vi "Old Auto Sequence.vi"() -> ()   [LabVIEW 2014]
uses:
  TypeDefs/SRE Enum.ctl
  <vilib>/Rock Robotics/Network Tables/SD Read Number.vi
  Support Code/Robot Global Data.vi
panel:
  in  "Direction":dbl=1.25 format="%#_13g"
  in  "Set To":dbl=-135.0 format="%#_13g"
  in  "Angle":dbl=-155.0 format="%#_13g"
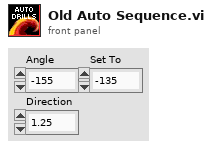
[diagram p1: front panel]
types:
  T1 = typedef "SRE Enum.ctl" = enum16{"Start", "Run", "End"}
  T2 = cluster{"Speed":dbl, "Direction":dbl, "Rotation":dbl}
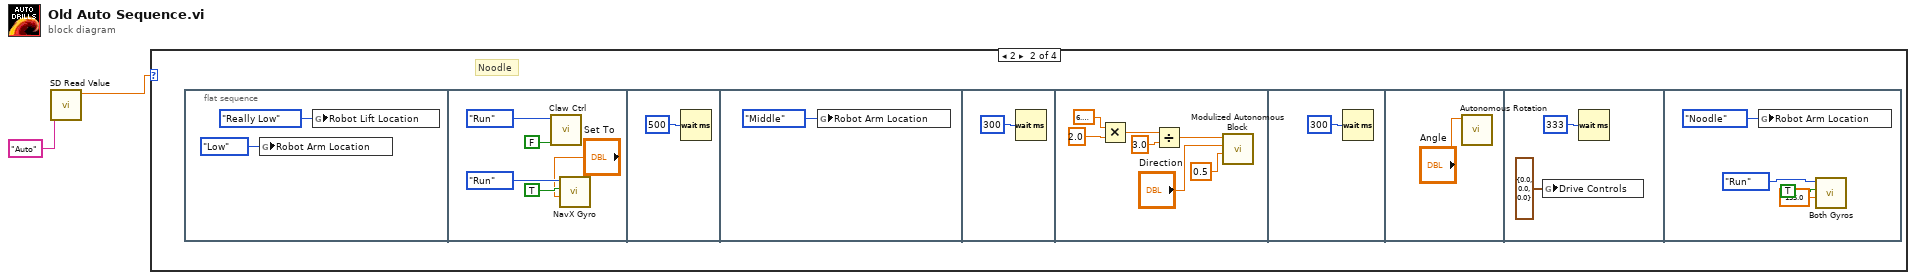
[diagram p0: block diagram]
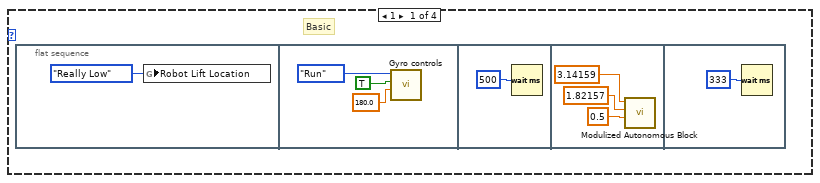
[diagram p2: hidden frame]
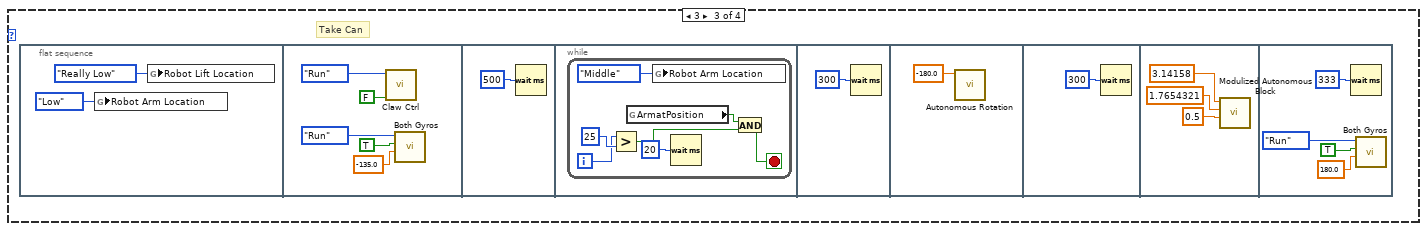
[diagram p3: hidden frame]
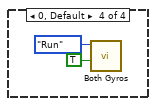
[diagram p4: hidden frame]
diagram:
  n1 = call-poly <vilib>:"SD Read Value.vi"("Name"="Auto") -> ("Numeric"=w1:dbl)  [unwired: 8 in, 2 out]
  n2 = case shown="2" w1 {
    frame 1 {
      # "Basic"
      n3 = flat-sequence {
        frame #0 {
          n4 = global write "Robot Global Data.vi" "Robot Lift Location"(enum16{"High", "Middle", "Low", "Really Low"}."Really Low" ("Robot Lift Location")) -> ()
        }
        frame #1 {
          n5 = call "Gyro controls.vi"("Set To"=180.0, "Reset"=TRUE, "Enum"=SRE_Enum."Run") -> ()  [unwired: 8 in, 1 out]
        }
        frame #2 {
          n6 = Wait (ms)(milliseconds to wait=u32 500) -> ()  [unwired: 1 out]
        }
        frame #3 {
          n7 = call "Modulized Autonomous Block.vi"("Power"=0.5, "run time in seconds"=1.82157 ("Direction"), "Direction"=3.14159) -> ()  [unwired: 8 in, 1 out]
        }
        frame #4 {
          n8 = Wait (ms)(milliseconds to wait=u32 333) -> ()  [unwired: 1 out]
        }
      }
    }
    frame 2 {
      # "Noodle"
      n9 = flat-sequence {
        frame #0 {
          n10 = global write "Robot Global Data.vi" "Robot Arm Location"(enum16{"High", "Middle", "Low", "Noodle"}."Low" ("Robot Arm Location")) -> ()
          n11 = global write "Robot Global Data.vi" "Robot Lift Location"(enum16{"High", "Middle", "Low", "Really Low"}."Really Low" ("Robot Lift Location")) -> ()
        }
        frame #1 {
          n12 = call "Claw Ctrl.vi"("Open/Close"=FALSE, "Enum"=SRE_Enum."Run") -> ()  [unwired: 10 in]
          n13 = call "NavX Gyro.vi"("Set To"="Set To", "Reset"=TRUE, "Enum"=SRE_Enum."Run") -> ()  [unwired: 7 in, 2 out]
        }
        frame #2 {
          n14 = Wait (ms)(milliseconds to wait=u32 500) -> ()  [unwired: 1 out]
        }
        frame #3 {
          n15 = global write "Robot Global Data.vi" "Robot Arm Location"(enum16{"High", "Middle", "Low", "Noodle"}."Middle" ("Robot Arm Location")) -> ()
        }
        frame #4 {
          n16 = Wait (ms)(milliseconds to wait=u32 300) -> ()  [unwired: 1 out]
        }
        frame #5 {
          n17 = Multiply(x=6.283185307179586, y=2.0) -> (x*y=w25:dbl)
          n18 = Divide(x=w25, y=3.0) -> (x/y=w23:dbl)
          n19 = call "Modulized Autonomous Block.vi"("Power"=0.5, "run time in seconds"="Direction", "Direction"=w23) -> ()  [unwired: 8 in, 1 out]
        }
        frame #6 {
          n20 = Wait (ms)(milliseconds to wait=u32 300) -> ()  [unwired: 1 out]
        }
        frame #7 {
          n21 = call "Autonomous Rotation.vi"("Angle"="Angle") -> ()  [unwired: 11 in]
        }
        frame #8 {
          n22 = global write "Robot Global Data.vi" "Drive Controls"(T2 {"Speed"=0.0, "Direction"=0.0, "Rotation"=0.0} ("Drive Controls")) -> ()
          n23 = Wait (ms)(milliseconds to wait=u32 333) -> ()  [unwired: 1 out]
        }
        frame #9 {
          n24 = global write "Robot Global Data.vi" "Robot Arm Location"(enum16{"High", "Middle", "Low", "Noodle"}."Noodle" ("Robot Arm Location")) -> ()
          n25 = call "Both Gyros.vi"("Set To"=-155.0, "Reset"=TRUE, "Enum"=SRE_Enum."Run") -> ()  [unwired: 8 in, 1 out]
        }
      }
    }
    frame 3 {
      # "Take Can"
      n26 = flat-sequence {
        frame #0 {
          n27 = global write "Robot Global Data.vi" "Robot Arm Location"(enum16{"High", "Middle", "Low", "Noodle"}."Low" ("Robot Arm Location")) -> ()
          n28 = global write "Robot Global Data.vi" "Robot Lift Location"(enum16{"High", "Middle", "Low", "Really Low"}."Really Low" ("Robot Lift Location")) -> ()
        }
        frame #1 {
          n29 = call "Claw Ctrl.vi"("Open/Close"=FALSE, "Enum"=SRE_Enum."Run") -> ()  [unwired: 10 in]
          n30 = call "Both Gyros.vi"("Set To"=-135.0, "Reset"=TRUE, "Enum"=SRE_Enum."Run") -> ()  [unwired: 8 in, 1 out]
        }
        frame #2 {
          n31 = Wait (ms)(milliseconds to wait=u32 500) -> ()  [unwired: 1 out]
        }
        frame #3 {
          n32 = while {
            i -> [w45]
            stop <- w49 stop-if-true
            n33 = Greater?(x=w45, y=25 ("x")) -> (0:w47:bool)
            n34 = global read "Robot Global Data.vi" "ArmatPosition"() -> (w48:bool)
            n35 = global write "Robot Global Data.vi" "Robot Arm Location"(enum16{"High", "Middle", "Low", "Noodle"}."Middle" ("Robot Arm Location")) -> ()
            n36 = Wait (ms)(milliseconds to wait=u32 20) -> ()  [unwired: 1 out]
            n37 = And(x=w48, y=w47) -> (x .and. y?=w49:bool)
          }
        }
        frame #4 {
          n38 = Wait (ms)(milliseconds to wait=u32 300) -> ()  [unwired: 1 out]
        }
        frame #5 {
          n39 = call "Autonomous Rotation.vi"("Angle"=-180.0) -> ()  [unwired: 11 in]
        }
        frame #6 {
          n40 = Wait (ms)(milliseconds to wait=u32 300) -> ()  [unwired: 1 out]
        }
        frame #7 {
          n41 = call "Modulized Autonomous Block.vi"("Power"=0.5, "run time in seconds"=1.7654321 ("Direction"), "Direction"=3.14158) -> ()  [unwired: 8 in, 1 out]
        }
        frame #8 {
          n42 = Wait (ms)(milliseconds to wait=u32 333) -> ()  [unwired: 1 out]
          n43 = call "Both Gyros.vi"("Set To"=180.0, "Reset"=TRUE, "Enum"=SRE_Enum."Run") -> ()  [unwired: 8 in, 1 out]
        }
      }
    }
    frame 0, Default {
      n44 = call "Both Gyros.vi"("Reset"=TRUE, "Enum"=SRE_Enum."Run") -> ()  [unwired: 9 in, 1 out]
    }
  }
